vi "Send Register.vi"(7 "Event":refnum<class "Event.lvclass">, 8 "Error In":errorcluster, 9 "Event Handler":refnum<class "Event Generated Msg.lvclass">, 10 "Registrant Address":refnum<class "Message Enqueuer.lvclass">, 11 "Event Source Address":refnum<class "Message Enqueuer.lvclass">) -> (0 "Error Out":errorcluster, 3 "Event Source Address Out":refnum<class "Message Enqueuer.lvclass">)   [LabVIEW 2016, in "Event Source.lvlib" / "Register Msg.lvclass"]
doc: "Send Register for event message to the Event Source Actor. This adds the Event for which the registrant wants to listen to and associates with it the Zero Coupling message for handling the event and the registrants return address."
uses:
  Register Msg.lvclass
  <vilib>/ActorFramework/Message Enqueuer/Message Enqueuer.lvclass
  Event/Event.lvclass
  Event Generated Msg/Event Generated Msg.lvclass
  C:/Program Files (x86)/National Instruments/LabVIEW 2016/vi.lib/ActorFramework/Message/Message.lvclass
  Register Msg.lvclass/Register Msg.ctl
  <vilib>/ActorFramework/Message Enqueuer/Message Enqueuer.lvclass/Message Enqueuer.ctl
  <vilib>/ActorFramework/Message Priority Queue/Priority Enqueue.vi
  <resource>/AFDebug/Generate Trace for Message.vi
  <vilib>/Utility/LVClass/Get LV Class Name.vi
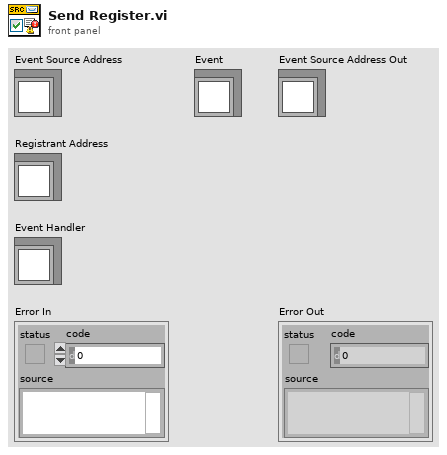
[diagram p1: front panel]
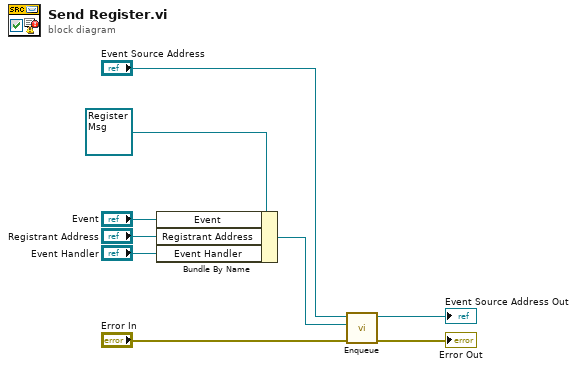
[diagram p0: block diagram]
diagram:
  n1 = Bundle By Name(cluster=refnum<class "Register Msg.lvclass"> refnum ("Message Type"), "Event"="Event", "Registrant Address"="Registrant Address", "Event Handler"="Event Handler") -> (w5:refnum<class "Register Msg.lvclass">)
  n2 = call <vilib>:"Enqueue.vi"("error in (no error)"="Error In", "Message"=w5, "Message Enqueuer in"="Event Source Address") -> ("error out"=→"Error Out":errorcluster, "Message Enqueuer out"=→"Event Source Address Out":refnum<class "Message Enqueuer.lvclass">)  [unwired: 7 in]
